vi "Data Rescue.vi"(2 "Separator":string, 3 "Input String":string) -> (0 "Humidity (%)":fxp<+/-,64,32>, 1 "Temperature":fxp<+/-,64,32>)   [LabVIEW 2020]
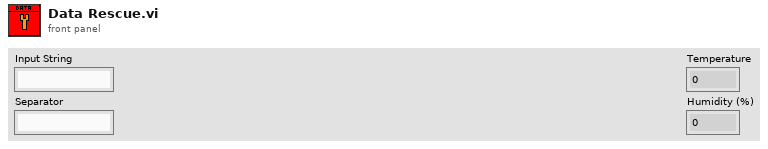
[diagram p1: front panel]
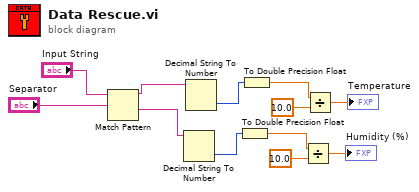
[diagram p0: block diagram]
diagram:
  n1 = Match Pattern(string="Input String", regular expression="Separator") -> (before substring=w11:string, after substring=w12:string)  [unwired: 1 in, 2 out]
  n2 = Decimal String To Number(string=w12) -> (number=w7:i32)  [unwired: 2 in, 1 out]
  n3 = Decimal String To Number(string=w11) -> (number=w10:i32)  [unwired: 2 in, 1 out]
  n4 = To Double Precision Float(number=w7) -> (double precision float=w6:dbl)
  n5 = To Double Precision Float(number=w10) -> (double precision float=w9:dbl)
  n6 = Divide(x=w6, y=10.0) -> (x/y=→"Humidity (%)":dbl)
  n7 = Divide(x=w9, y=10.0) -> (x/y=→"Temperature":dbl)
